vi "Replace SubWaveform.vi"(8 "error in (no error)":errorcluster, 9 "Index":i32, 10 "Waveform.lvclass":refnum<class "Waveform.lvclass">, 11 "Composite Waveform in":refnum<class "Composite Waveform.lvclass">) -> (0 "error out":errorcluster, 3 "Composite Waveform out":refnum<class "Composite Waveform.lvclass">)   [LabVIEW 2016, in "Composite Waveform.lvclass"]
uses:
  Composite Waveform.lvclass
  Waveform/Waveform.lvclass
  Composite Waveform.lvclass/Composite Waveform.ctl
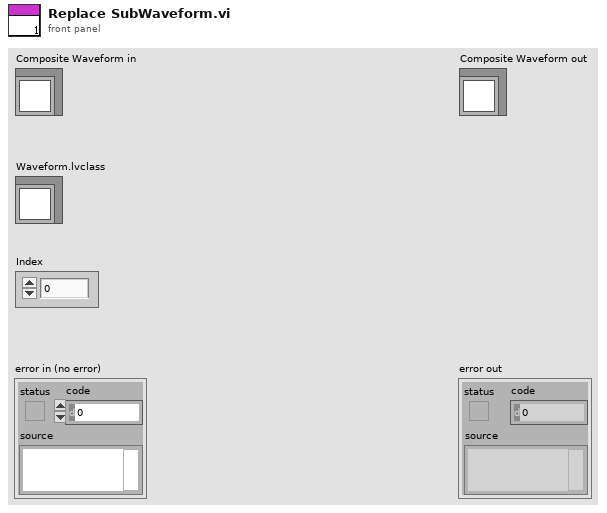
[diagram p1: front panel]
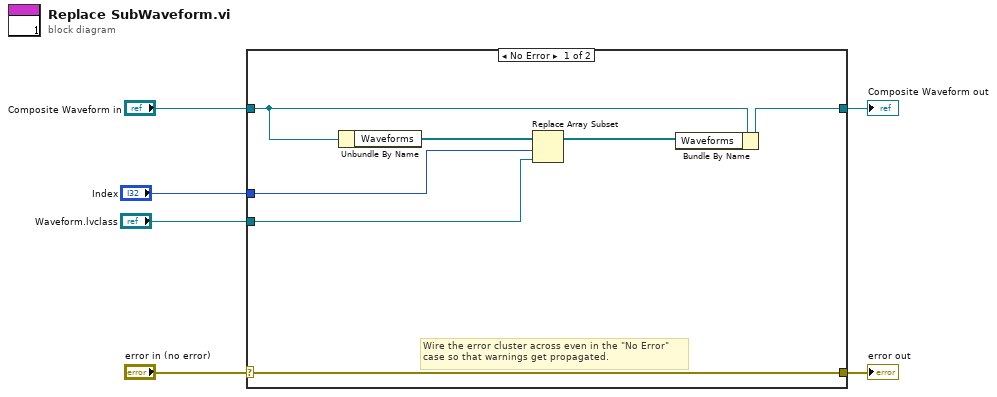
[diagram p0: block diagram]
diagram:
  n1 = case shown="No Error" "error in (no error)" {
    selector: "error in (no error)" -> [w13 w15]
    tunnel: [w13 w15] -> w5
    tunnel: [w11 w14] -> w3
    tunnel: "Composite Waveform in" -> [w12 w14]
    tunnel: "Waveform.lvclass" -> [w8 _]
    tunnel: "Index" -> [w7 _]
    frame No Error {
      # "Wire the error cluster across even in the \"No Error\"\ncase so that warnings get propagated."
      n2 = Unbundle By Name(w12) -> ("Waveforms"=w10:refnum<class "Waveform.lvclass">[])
      n3 = Replace Array Subset(array=w10, new element=w8, index=w7) -> (w9:refnum<class "Waveform.lvclass">[])
      n4 = Bundle By Name(cluster=w12, "Waveforms"=w9) -> (w11:refnum<class "Composite Waveform.lvclass">)
    }
    frame Error {
    }
  }
  "error out" <- w5
  "Composite Waveform out" <- w3
